vi "Get Image Data.vi"(4 "Image Info Queu":refnum<queue>[](array[refnum]), 7 "serial channel display parameters":refnum<notifier>, 8 "error in (no error)":errorcluster, 9 "fpga interface in":refnum<k20>, 10 "Acquisition Stopped Notifier":refnum<notifier>, 11 "Measure Call Context in":refnum<class "Measure Call Context.lvclass">) -> (0 "error out":errorcluster)   [LabVIEW 2025, in "Automotive Vision.lvclass"]
uses:
  Automotive Vision.lvclass
  <vilib>/Plug-In SDKs/Measurements/Measure Call Context/Measure Call Context.lvclass
  Automotive Vision.lvclass/Automotive Vision.ctl
  <vilib>/vision/Image Controls.llb/IMAQ Image.ctl
  deps/NI148X/Getting Started/Host/Common/Types/RAW Interpretation for Display.ctl
  deps/NI148X/Getting Started/Host/Common/GettingStarted_Common_148X_Host.lvlib
  deps/NI148X/Getting Started/Host/Common/Types/Serial Channel Display Parameters.ctl
  <instrlib>/FlexRIO/CSI-2/v2/Common/Types/LLP Data Type.ctl
  <instrlib>/FlexRIO/CSI-2/v2/Common/NI CSI-2 API Common v2.lvlib
  deps/NI148X/Getting Started/FPGA/Common/Types/Image Metadata.ctl
  deps/NI148X/Getting Started/FPGA/Common/GettingStarted_Common_148X_FPGA.lvlib
  Types/Image Info.ctl
  Types/Status Data.ctl
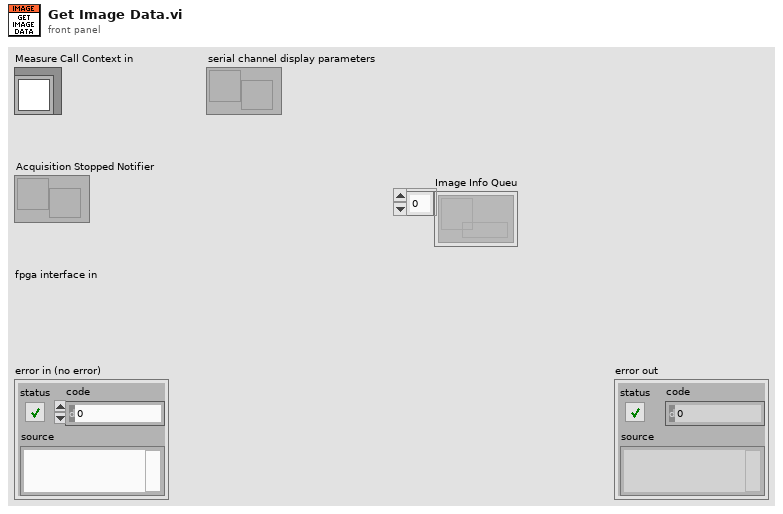
[diagram p1: front panel]
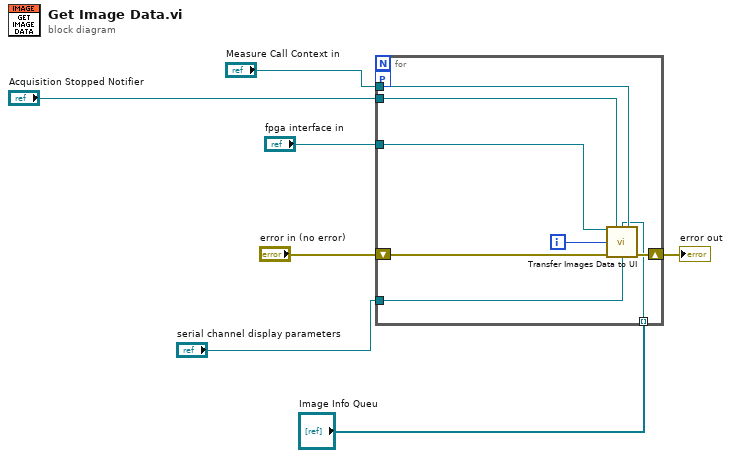
[diagram p0: block diagram]
diagram:
  n1 = for {
    tunnel: "fpga interface in" -> [w13]
    tunnel: "Acquisition Stopped Notifier" -> [w12]
    tunnel: "Measure Call Context in" -> [w11]
    tunnel: "serial channel display parameters" -> [w10]
    shift-right: [w15] -> w2
    shift-left: "error in (no error)" -> [w14]
    workers-P: _ -> [_]
    tunnel: "Image Info Queu" -> [w8] mode=indexing
    i -> [w9]
    n2 = call "Transfer Images Data to UI.vi"("fpga interface in"=w13, "'stop' notifier"=w12, "Image Info"=w8, "measure call context in"=w11, "display channel number"=w9, "error in"=w14, "raw display notifier"=w10) -> ("error out"=w15:errorcluster)  [unwired: 7 in, 1 out]
  }
  "error out" <- w2
